vi "ErrorHandlerFGV.vi"(7 "Command(CheckErrors)":enum16{"Initialize", "CheckErrors"}(ring)=enum."CheckErrors", 10 "Error In":errorcluster, 11 "MHL":refnum<queue>) -> (2 "Error Out":errorcluster)   [LabVIEW 2017, in "Server.lvlib" / "ErrorLogger.lvlib"]
doc: "This VI checks if an error occured. If yes, it sends the error in the MHL-Queue which forwards it to Error-Queue for further processing. The error is deleted afterwards.\nThe Error-Logger-Loop will then receive the error and decide what to do (propably shut down the Application)"
uses:
  ErrorLogger.lvlib
  Message Queue/MessageCluster.ctl
  Message Queue/EnqueueMessage(Single).vi
  Message Queue/Message Queue.lvlib
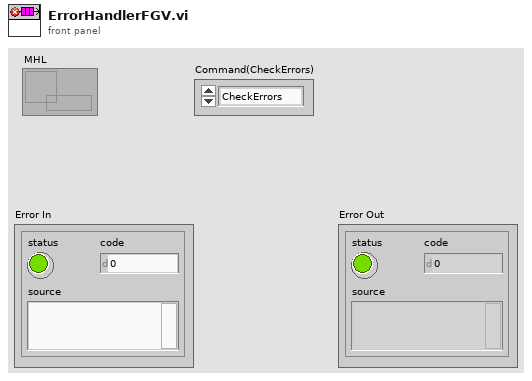
[diagram p1: front panel]
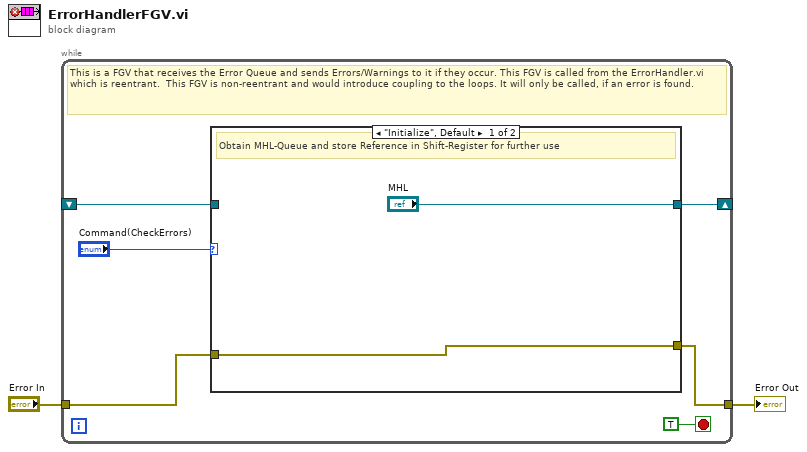
[diagram p0: block diagram]
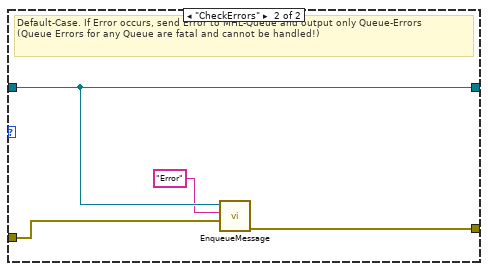
[diagram p2: hidden frame]
diagram:
  n1 = while {
    shift-right: [w6] -> _
    shift-left: _ -> [w7]
    tunnel: "Error In" -> [w4]
    tunnel: [w3] -> w1
    stop <- TRUE stop-if-true
    # "This is a FGV that receives the Error Queue and sends Errors/Warnings to it if they occur. This FGV is called from the ErrorHandler.vi which is reentrant.  This FGV is non-reentrant and would introduce coupling to the loops. It will only be called, if an error is found."
    n2 = case shown="\"Initialize\", Default" "Command(CheckErrors)" {
      tunnel: ["MHL" w13] -> w6
      tunnel: w7 -> [_ w13]
      tunnel: [w9 w14] -> w3
      tunnel: w4 -> [w9 w12]
      frame "Initialize", Default {
        # "Obtain MHL-Queue and store Reference in Shift-Register for further use"
      }
      frame "CheckErrors" {
        # "Default-Case. If Error occurs, send Error to MHL-Queue and output only Queue-Errors\n(Queue Errors for any Queue are fatal and cannot be handled!)"
        n3 = call-poly "EnqueueMessage.vi"("Message Data"=w12, "Message"="Error", "Message Queue"=w13) -> ("error out"=w14:errorcluster)  [unwired: 7 in, 1 out]
      }
    }
  }
  "Error Out" <- w1
